vi "Verify Built.vi"(8 "error in (no error)":errorcluster, 11 "Table Configuration in":refnum<class "Table Configuration.lvclass">) -> (0 "error out":errorcluster, 3 "Table Configuration out":refnum<class "Table Configuration.lvclass">)   [LabVIEW 2020, in "Table.lvlib" / "Table Configuration.lvclass"]
uses:
  Table Configuration.lvclass
  Table Configuration.lvclass/Table Configuration.ctl
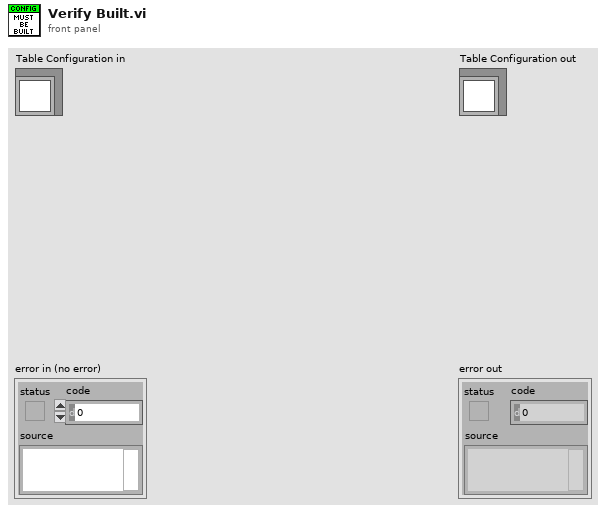
[diagram p1: front panel]
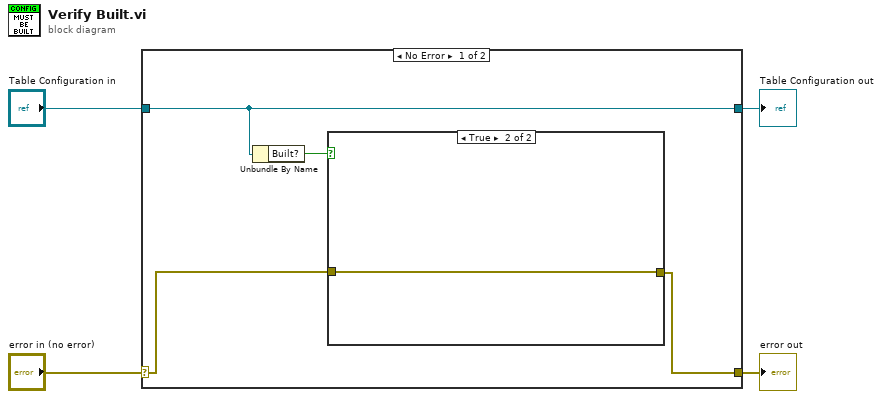
[diagram p0: block diagram]
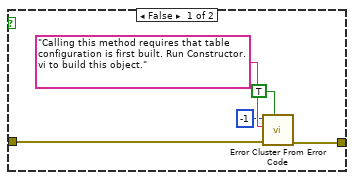
[diagram p2: hidden frame]
diagram:
  n1 = case shown="No Error" "error in (no error)" {
    selector: "error in (no error)" -> [w6 w16]
    tunnel: [w5 w16] -> w3
    tunnel: [w8 w15] -> w1
    tunnel: "Table Configuration in" -> [w8 w15]
    frame No Error {
      n2 = Unbundle By Name(w8) -> ("Built?"=w7:bool)
      n3 = case shown="True" w7 {
        tunnel: w6 -> [w10 w14]
        tunnel: [w9 w14] -> w5
        frame False {
          n4 = call <vilib>:"Error Cluster From Error Code.vi"("show call chain? (False)"=TRUE, "error in (no error)"=w10, "error message (\"\")"="Calling this method requires that table configuration is first built. Run Constructor.vi to build this object.", "error code (0)"=-1) -> ("error out"=w9:errorcluster)  [unwired: 5 in]
        }
        frame True {
        }
      }
    }
    frame Error {
    }
  }
  "error out" <- w3
  "Table Configuration out" <- w1
